vi "Mouse Up.vi"(8 "error in (no error)":errorcluster, 10 "Point":T1, 11 "Rectangle in":refnum<class "Triangle.lvclass">) -> (0 "error out":errorcluster, 3 "Rectangle out":refnum<class "Triangle.lvclass">)   [LabVIEW 2020, in "Triangle.lvclass"]
doc: "A method for specifying how a triangle reacts on a mouse up event"
uses:
  Triangle.lvclass
  D:/Git/Labview-Libraries/Tools/Drawing Tool Folder/Graphics Object/Graphics Object.lvclass
  D:/Git/Labview-Libraries/Tools/Drawing Tool Folder/Polygon/Polygon.lvclass
  <vilib>/Utility/miscctls.llb/LVPoint32TypeDef.ctl
  Line/Line.lvclass
  Graphics Object/Graphics Object.lvclass
  Polygon/Polygon.lvclass
panel:
  # "expressionflow.com"
  # "Copyright (c) 2008 Tomi Maila. All rights reserved."
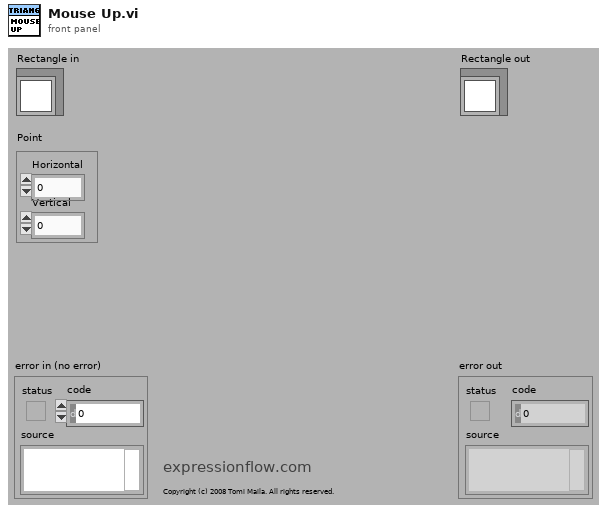
[diagram p1: front panel]
types:
  T1 = typedef "LVPoint32TypeDef.ctl" = cluster{"Horizontal":i32, "Vertical":i32}
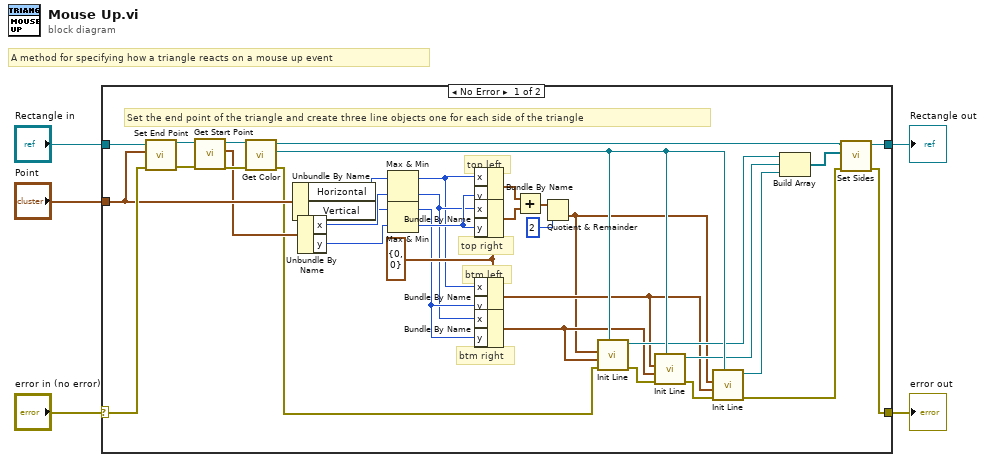
[diagram p0: block diagram]
diagram:
  # "A method for specifying how a triangle reacts on a mouse up event"
  n1 = case shown="No Error" "error in (no error)" {
    selector: "error in (no error)" -> [w32 w42]
    tunnel: [w17 w42] -> w4
    tunnel: [w20 w43] -> w2
    tunnel: "Rectangle in" -> [w33 w43]
    tunnel: "Point" -> [w27 _]
    frame No Error {
      w40 = cluster{"x":i16, "y":i16} {"x"=0, "y"=0} ("start point")
      # "Set the end point of the triangle and create three line objects one for each side of the triangle"
      # "btm right"
      # "btm left"
      # "top right"
      # "top left"
      n2 = call "Set End Point.vi"("error in (no error)"=w32, "end point (0,0)"=w27, "Graphics Object.lvclass in"=w33) -> ("error out"=w28:errorcluster, "Graphics Object.lvclass out"=w31:refnum<class "Triangle.lvclass">)  [unwired: 7 in]
      n3 = call "Get Start Point.vi"("error in (no error)"=w28, "Graphics Object.lvclass in"=w31) -> ("error out"=w29:errorcluster, "start point"=w26:cluster{"x":i16, "y":i16}, "Graphics Object.lvclass out"=w30:refnum<class "Triangle.lvclass">)  [unwired: 7 in]
      n4 = call-dynamic "Get Color.vi"("error in (no error)"=w29, "Geometric Object.lvclass in"=w30) -> ("error out"=w21:errorcluster, "Color.lvclass"=w34:refnum<class "Color.lvclass">, "Geometric Object.lvclass out"=w19:refnum<class "Triangle.lvclass">)  [unwired: 7 in]
      n5 = Unbundle By Name(w27) -> ("Horizontal"=w25:i32, "Vertical"=w23:i32)
      n6 = Unbundle By Name(w26) -> ("x"=w24:i16, "y"=w22:i16)
      n7 = Max & Min(x=w25, y=w24) -> (max(x,y)=w37:i32, min(x,y)=w38:i32)
      n8 = Max & Min(x=w23, y=w22) -> (max(x,y)=w39:i32, min(x,y)=w41:i32)
      n9 = Bundle By Name(cluster=w40, "x"=w37, "y"=w41) -> (w12:cluster{"x":i16, "y":i16})
      n10 = Bundle By Name(cluster=w40, "x"=w38, "y"=w41) -> (w11:cluster{"x":i16, "y":i16})
      n11 = Bundle By Name(cluster=w40, "x"=w37, "y"=w39) -> (w8:cluster{"x":i16, "y":i16})
      n12 = Bundle By Name(cluster=w40, "x"=w38, "y"=w39) -> (w7:cluster{"x":i16, "y":i16})
      n13 = Add(x=w12, y=w11) -> (x+y=w10:cluster{"x":i16, "y":i16})
      n14 = Quotient & Remainder(x=w10, y=i16 2) -> (floor(x/y)=w6:cluster{"x":i16, "y":i16})  [unwired: 1 out]
      n15 = call "Init Line.vi"("Color (RGB black)"=w34, "error in (no error)"=w21, "end point (0,0)"=w7, "start point (0,0)"=w6) -> ("error out"=w35:errorcluster, "Line out"=w16:refnum<class "Line.lvclass">)  [unwired: 6 in]
      n16 = call "Init Line.vi"("Color (RGB black)"=w34, "error in (no error)"=w35, "end point (0,0)"=w7, "start point (0,0)"=w8) -> ("error out"=w36:errorcluster, "Line out"=w15:refnum<class "Line.lvclass">)  [unwired: 6 in]
      n17 = call "Init Line.vi"("Color (RGB black)"=w34, "error in (no error)"=w36, "end point (0,0)"=w8, "start point (0,0)"=w6) -> ("error out"=w13:errorcluster, "Line out"=w14:refnum<class "Line.lvclass">)  [unwired: 6 in]
      n18 = Build Array(w16, w15, w14) -> (w18:refnum<class "Line.lvclass">[])
      n19 = call "Set Sides.vi"("error in (no error)"=w13, "Sides"=w18, "Polygon.lvclass in"=w19) -> ("error out"=w17:errorcluster, "Polygon.lvclass out"=w20:refnum<class "Triangle.lvclass">)  [unwired: 7 in]
    }
    frame Error {
    }
  }
  "error out" <- w4
  "Rectangle out" <- w2
